vi "chakan.vi"() -> ()   [LabVIEW 2012]
panel:
  out "错误信息":string="VOLT 1"
  out "存储器中的波形":string="VOLT 1"
  out "error out":errorcluster
  in  "串口参数设置":enum32{"常用设置", "不常用的"}(tab)
  in  "termination char\n(0xA = '\\n' = LF)":u8=10 caption="EOL字串-LF" format="%.0x"
  in  "flow control":u16(ring) caption="流量控制" items=["None"=0, "XON/XOFF"=1, "RTS/CTS"=2, "DTR/DSR"=4]
  in  "data bits":u16=8 caption="数据位" min=5 max=8 step=1
  in  "stop bits":u16(ring)=10 caption="停止位" items=["1.0"=10, "1.5"=15, "2.0"=20]
  in  "parity":u16(ring) caption="奇偶校验" items=["None", "Odd", "Even", "Mark", "Space"]
  in  "baud rate":u32=9600 caption="波特率"
  in  "VISA resource name":refnum<visa-resource-name>="COM1" caption="端口号"
  in  "timeout (ms)":u32=10000
  in  "XON Character":u8=17 format="%.0x"
  in  "XOFF Character":u8=19 format="%.0x"
  in  "Input buffer size":u32=4096 caption="输入缓冲区大小"
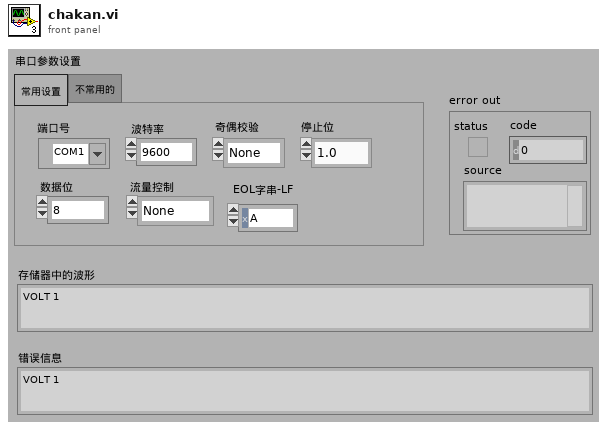
[diagram p1: front panel]
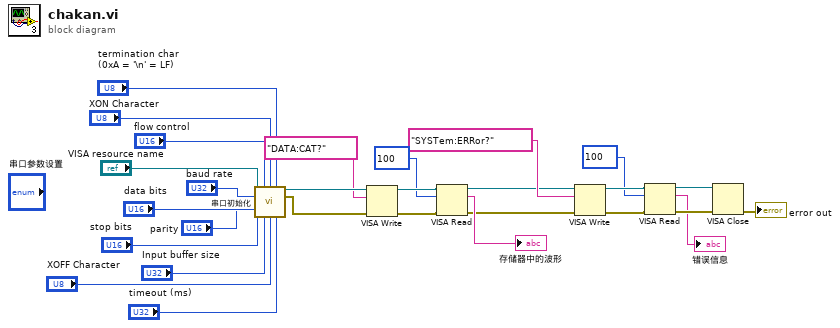
[diagram p0: block diagram]
diagram:
  n1 = call "串口初始化.vi"("VISA resource name"="VISA resource name", "flow control"="flow control", "XON Character"="XON Character", "termination char\n(0xA = '\\n' = LF)"="termination char\n(0xA = '\\n' = LF)", "baud rate"="baud rate", "data bits"="data bits", "parity"="parity", "stop bits"="stop bits", "Input buffer size"="Input buffer size", "XOFF Character"="XOFF Character", "timeout (ms)"="timeout (ms)") -> ("VISA resource name out"=w17:refnum<visa-resource-name>, "错误输出"=w15:errorcluster)  [unwired: 3 in]
  n2 = VISA Write(VISA resource name=w17, write buffer="DATA:CAT?" ("写入缓冲区"), error in (no error)=w15) -> (VISA resource name out=w13:refnum<visa-resource-name>, error out=w12:errorcluster)  [unwired: 1 out]
  n3 = VISA Read(VISA resource name=w13, byte count=u32 100 ("字节总数"), error in (no error)=w12) -> (VISA resource name out=w5:refnum<visa-resource-name>, read buffer=→"存储器中的波形":string, error out=w4:errorcluster)  [unwired: 1 out]
  n4 = VISA Write(VISA resource name=w5, write buffer="SYSTem:ERRor?" ("写入缓冲区"), error in (no error)=w4) -> (VISA resource name out=w8:refnum<visa-resource-name>, error out=w7:errorcluster)  [unwired: 1 out]
  n5 = VISA Read(VISA resource name=w8, byte count=u32 100 ("字节总数"), error in (no error)=w7) -> (VISA resource name out=w3:refnum<visa-resource-name>, read buffer=→"错误信息":string, error out=w2:errorcluster)  [unwired: 1 out]
  n6 = VISA Close(VISA resource name=w3, error in (no error)=w2) -> (error out=→"error out":errorcluster)
